vi "Simple Resolve Example.vi"() -> ()   [LabVIEW 2020, in "Futures-Examples.lvlib"]
uses:
  Futures-Examples.lvlib
  Promises/Future/Future.lvclass
  a5ae5b97-93ec-4ffd-8608-d35cef35f14e.vi
  c1f70840-660b-49b6-8a5a-babbc3cf0a41.vi
  DoubleValue/DoubleValue.lvclass
panel:
  in  "Timeout mS":i32=2000
  out "Value":dbl
  out "Error":errorcluster
  out "Milliseconds":u32
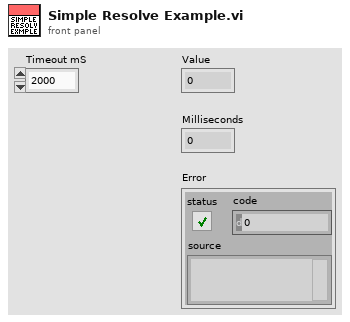
[diagram p1: front panel]
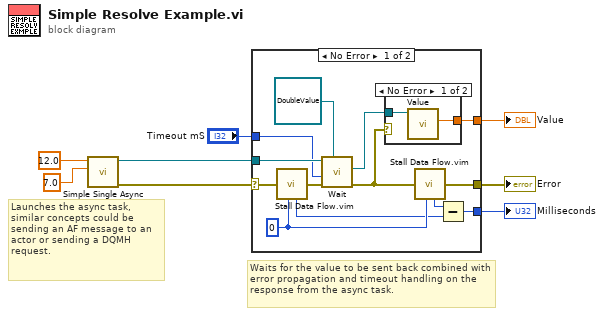
[diagram p0: block diagram]
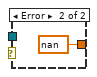
[diagram p2: hidden frame]
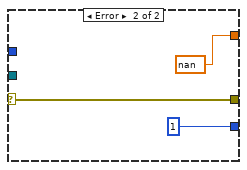
[diagram p3: hidden frame]
diagram:
  # "Waits for the value to be sent back combined with error propagation and timeout handling on the response from the async task."
  # "Launches the async task, similar concepts could be sending an AF message to an actor or sending a DQMH request."
  n1 = call "Simple Single Async.vi"("B"=7.0 ("A"), "A"=12.0) -> ("error out"=w5:errorcluster, "Future"=w6:refnum<class "Future.lvclass">)  [unwired: 8 in]
  n2 = case shown="No Error" w5 {
    selector: w5 -> [w20 w27]
    tunnel: w6 -> [w21 _]
    tunnel: [w15 u32 1] -> w4
    tunnel: [w14 w27] -> w3
    tunnel: [w11 nan ("Value")] -> w2
    tunnel: "Timeout mS" -> [w10 _]
    frame No Error {
      w18 = u32 0 ("milliseconds to wait")
      n3 = call "Stall Data Flow.vim"("value in"=w20, "milliseconds to wait"=w18) -> ("millisecond timer value"=w16:u32, "value out"=w19:errorcluster)
      n4 = call "Wait.vi"("Result Type"=refnum<class "DoubleValue.lvclass"> refnum ("Futures-Examples.lvlib:DoubleValue.lvclass"), "error in (no error)"=w19, "Timeout mS (-1)"=w10, "Future in"=w21) -> ("error out"=w9:errorcluster, "Result"=w12:refnum<class "DoubleValue.lvclass">)  [unwired: 6 in]
      n5 = case shown="No Error" w9 {
        tunnel: w12 -> [w23 _]
        tunnel: [w22 nan ("Value")] -> w11
        frame No Error {
          n6 = call "Value.vi"("DoubleValue in"=w23) -> ("Value"=w22:dbl)  [unwired: 10 in]
        }
        frame Error {
        }
      }
      n7 = call "Stall Data Flow.vim"("value in"=w9, "milliseconds to wait"=w18) -> ("millisecond timer value"=w17:u32, "value out"=w14:errorcluster)
      n8 = Subtract(x=w17, y=w16) -> (x-y=w15:u32)
    }
    frame Error {
    }
  }
  "Milliseconds" <- w4
  "Error" <- w3
  "Value" <- w2
